vi "Get Array Value at Index - Known Type.vi"(6 "Get Value as JSON Tree? (F)":bool, 8 "error in (no error)":errorcluster, 10 "Index":i32, 11 "JSON Tree In (JSON Array)":variant) -> (0 "error out":errorcluster, 1 "is JSON Null?":bool, 2 "Value":variant, 3 "JSON Tree Out Passthrough":variant, 5 "JSON Compatible Type":T1=enum."Unknown", 7 "JSON Type":T2=enum."Unknown")   [LabVIEW 2011, in "i3-json.lvlib"]
doc: "Use this template to build a VI to use as a subVI."
uses:
  i3-json.lvlib
  JSON Types/JSON Type.ctl
  JSON Types/JSON Compatible Type.ctl
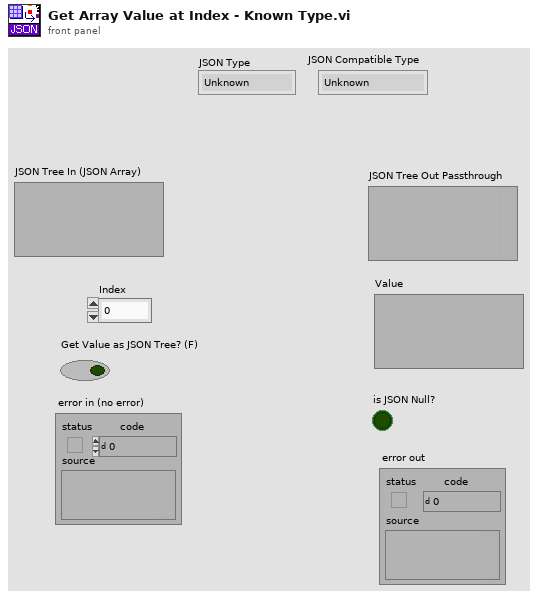
[diagram p1: front panel]
types:
  T1 = typedef "i3-json.lvlib/JSON Compatible Type.ctl" = enum16{"1D Double Array", "1D String Array", "1D Boolean Array", "Unknown"}
  T2 = typedef "i3-json.lvlib/JSON Type.ctl" = enum8{"JSON Compatible", "JSON Array", "JSON Object", "JSON Null", "Double", "String", "Boolean", "Unknown", "Data JSON string"}
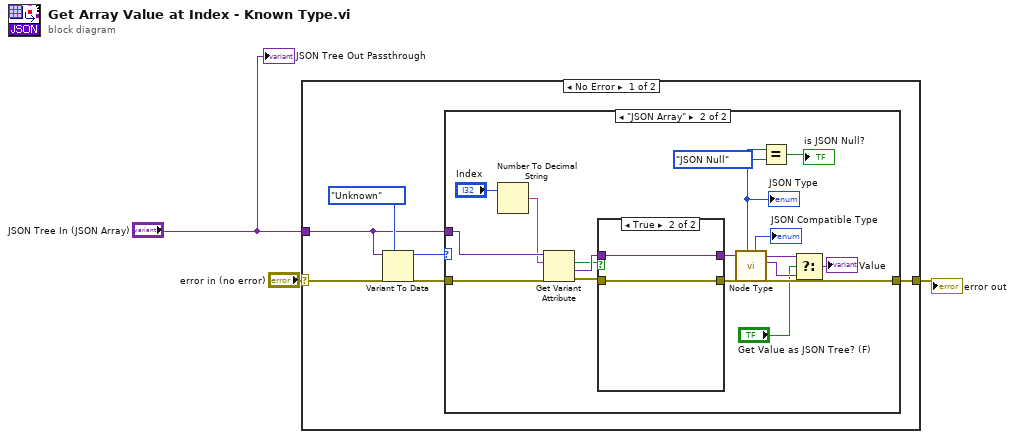
[diagram p0: block diagram]
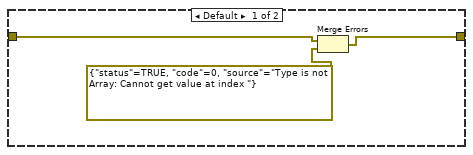
[diagram p2: hidden frame]
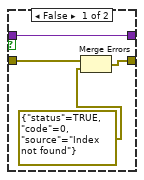
[diagram p3: hidden frame]
diagram:
  n1 = case shown="No Error" "error in (no error)" {
    selector: "error in (no error)" -> [w9 w37]
    tunnel: [w5 w37] -> w2
    tunnel: "JSON Tree In (JSON Array)" -> [w4 _]
    frame No Error {
      n2 = Variant To Data(error in=w9, type=JSON_Type."Unknown" ("JSON Type"), Variant=w4) -> (data=w6:T2, error out=w7:errorcluster)
      n3 = case shown="\"JSON Array\"" w6 {
        tunnel: w7 -> [w11 w30]
        tunnel: w4 -> [_ w28]
        tunnel: [w10 w26] -> w5
        frame Default {
          n4 = Merge Errors(w11, errorcluster {"status"=TRUE, "code"=0, "source"="Type is not Array: Cannot get value at index "} ("error out")) -> (w10:errorcluster)
        }
        frame "JSON Array" {
          n5 = Number To Decimal String(number="Index") -> (decimal integer string=w27:string)  [unwired: 1 in]
          n6 = Get Variant Attribute(Variant=w28, name=w27, error in=w30) -> (found=w20:bool, value=w22:variant, error out=w21:errorcluster)  [unwired: 1 in, 1 out]
          n7 = case shown="True" w20 {
            tunnel: w21 -> [w32 w36]
            tunnel: [w33 w36] -> w24
            tunnel: w22 -> [w34 w35]
            tunnel: [w34 w35] -> w23
            frame False {
              n8 = Merge Errors(w32, errorcluster {"status"=TRUE, "code"=0, "source"="Index not found"} ("error out")) -> (w33:errorcluster)
            }
            frame True {
            }
          }
          n9 = call "Node Type.vi"("error in (no error)"=w24, "JSON Tree In"=w23) -> ("error out"=w26:errorcluster, "Value"=w14:variant, "JSON Tree Passthrough"=w15:variant, "JSON Compatible Type"=→"JSON Compatible Type":T1, "JSON Type"=w18:T2)  [unwired: 5 in]
          "JSON Type" <- w18
          n10 = Equal?(x=w18, y=JSON_Type."JSON Null") -> (x = y?=→"is JSON Null?":bool)
          n11 = Select(t=w15, s="Get Value as JSON Tree? (F)", f=w14) -> (s? t:f=→"Value":variant)
        }
      }
    }
    frame Error {
    }
  }
  "error out" <- w2
  "JSON Tree Out Passthrough" <- "JSON Tree In (JSON Array)"
